vi "Remove Channel.vi"(8 "error in":errorcluster, 10 "name":string, 11 "transfer":T5={"core"={"name"="Transfer"}, "component settings"=[], "channels"=[]} {"channels"."core"."string offset" format="%d bytes"}) -> (0 "error out":errorcluster, 1 "found?":bool, 2 "removed channel":T1={"core"={"name"="Channel", "units"="V", "engine data type"=enum."DBL", "string data type"=enum."DBL", "string offset"=0}, "component settings"=[]} {"core"."string offset" format="%d bytes"}, 3 "transfer out":T5={"core"={"name"="Transfer"}, "component settings"=[], "channels"=[]} {"channels"."core"."string offset" format="%d bytes"})   [LabVIEW 2020, in "DSF Configuration API.lvlib"]
uses:
  DSF Configuration API.lvlib
  Includes/DSF Core.lvlibp/Typedefs/DSF Engine Transfer Configuration.ctl
  Includes/DSF Core.lvlibp/Typedefs/Core Transfer Configuration.ctl
  Includes/DSF Core.lvlibp/Typedefs/DSF Settings Info.ctl
  Includes/DSF Core.lvlibp/Typedefs/DSF Engine Channel Configuration.ctl
  Includes/DSF Core.lvlibp/Typedefs/Core Channel Configuration.ctl
  Includes/DSF Core.lvlibp/Typedefs/DSF Data Type.ctl
  Includes/DSF Core.lvlibp/Classes/Configuration/Core/Transfer/Transfer Configuration.lvclass
  Includes/DSF Core.lvlibp
  Includes/DSF Core.lvlibp/Classes/Configuration/Core/Channel/Channel Configuration.lvclass
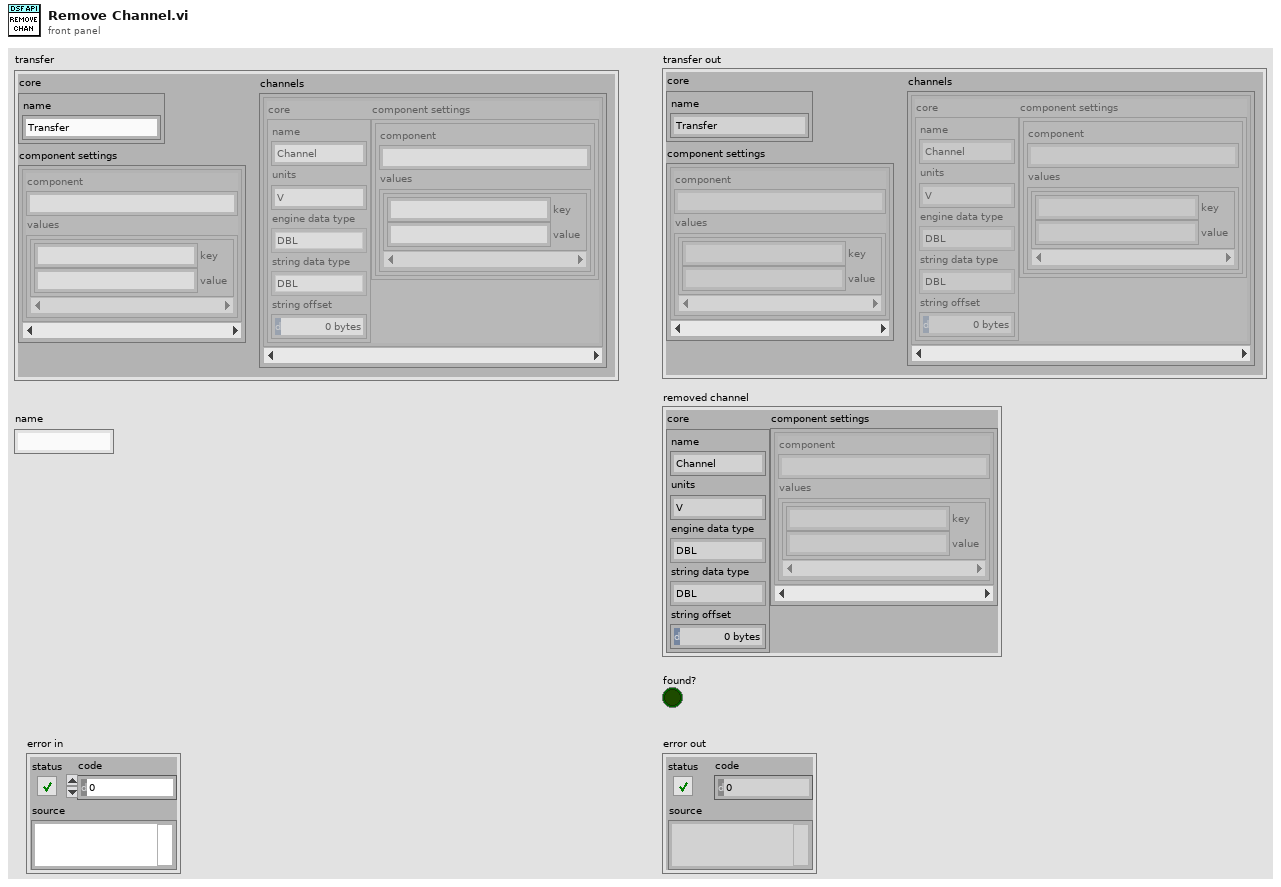
[diagram p1: front panel]
types:
  T1 = typedef "DSF Core.lvlibp/DSF Engine Channel Configuration.ctl" = cluster{"core":T2, "component settings":T4[]}
  T2 = typedef "DSF Core.lvlibp/Channel Configuration.lvclass/Core Channel Configuration.ctl" = cluster{"name":string, "units":string, "engine data type":T3, "string data type":T3, "string offset":u64}
  T3 = typedef "DSF Core.lvlibp/DSF Data Type.ctl" = enum8{"Bool", "SGL", "DBL", "I8", "I16", "I32", "I64", "U8", "U16", "U32", "U64"}
  T4 = typedef "DSF Core.lvlibp/DSF Settings Info.ctl" = cluster{"component":string, "values":cluster{"key":string, "value":string}[]}
  T5 = typedef "DSF Core.lvlibp/DSF Engine Transfer Configuration.ctl" = cluster{"core":T6, "component settings":T4[], "channels":T1[]}
  T6 = typedef "DSF Core.lvlibp/Transfer Configuration.lvclass/Core Transfer Configuration.ctl" = cluster{"name":string}
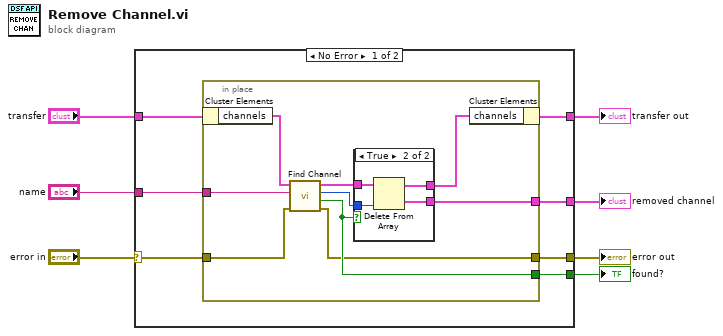
[diagram p0: block diagram]
diagram:
  n1 = case shown="No Error" "error in" {
    selector: "error in" -> [w11 w29]
    tunnel: "transfer" -> [w13 w30]
    tunnel: "name" -> [w14 _]
    tunnel: [w12 w30] -> w4
    tunnel: [w10 _] -> w3
    tunnel: [w9 _] -> w2
    tunnel: [w8 w29] -> w1
    frame No Error {
      n2 = in-place {
        in-place-border: w14 -> [w23]
        in-place-border: w11 -> [w18]
        in-place-border: [w17] -> w10
        in-place-border: [w16] -> w9
        in-place-border: [w15] -> w8
        n3 = in-place-cluster #1(w13) -> ("channels"=w21:T1[])
        n4 = call "Find Channel.vi"("error in"=w18, "name"=w23, "channels"=w21) -> ("error out"=w15:errorcluster, "found?"=w16:bool, "index"=w20:i32, "channels out"=w22:T1[])  [unwired: 5 in]
        n5 = case shown="True" w16 {
          tunnel: w22 -> [w24 w28]
          tunnel: w20 -> [_ w27]
          tunnel: [w24 w26] -> w19
          tunnel: [_ w25] -> w17
          frame False {
          }
          frame True {
            n6 = Delete From Array(array=w28, index=w27) -> (deleted portion=w25:T1, array with subset deleted=w26:T1[])  [unwired: 1 in]
          }
        }
        n7 = in-place-cluster #1("channels"=w19) -> (w12:T5)
      }
    }
    frame Error {
    }
  }
  "error out" <- w1
  "transfer out" <- w4
  "removed channel" <- w3
  "found?" <- w2
